vi "setStart_trigger.vi"(8 "error in (no error)":errorcluster, 10 "start_trigger":string, 11 "CameraAcquisitor.lvclass in":refnum<class "CameraAcquisitor.lvclass">) -> (0 "error out":errorcluster, 3 "CameraAcquisitor.lvclass out":refnum<class "CameraAcquisitor.lvclass">)   [LabVIEW 2011, in "Hardware.lvlib" / "Channels.lvlib" / "CameraAcquisitor.lvclass"]
uses:
  CameraAcquisitor.lvclass
  CameraAcquisitor.lvclass/CameraAcquisitor.ctl
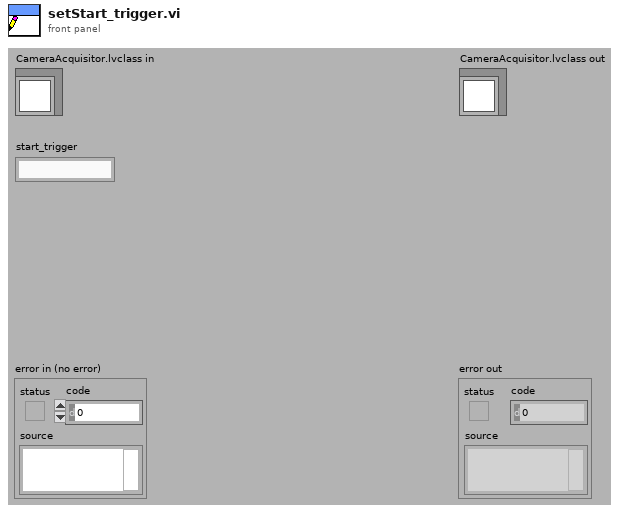
[diagram p1: front panel]
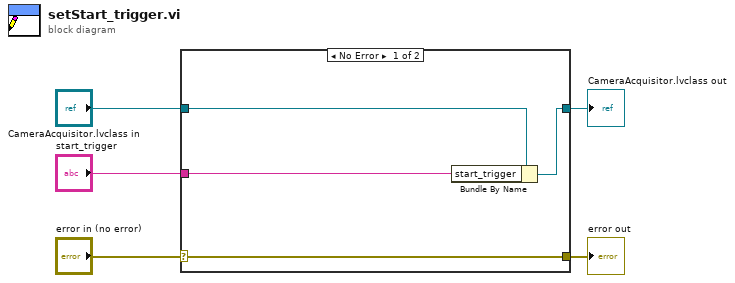
[diagram p0: block diagram]
diagram:
  n1 = case shown="No Error" "error in (no error)" {
    selector: "error in (no error)" -> [w9 w10]
    tunnel: [w9 w10] -> w4
    tunnel: [w7 w11] -> w2
    tunnel: "CameraAcquisitor.lvclass in" -> [w8 w11]
    tunnel: "start_trigger" -> [w6 _]
    frame No Error {
      n2 = Bundle By Name(cluster=w8, "start_trigger"=w6) -> (w7:refnum<class "CameraAcquisitor.lvclass">)
    }
    frame Error {
    }
  }
  "error out" <- w4
  "CameraAcquisitor.lvclass out" <- w2
